vi "LS370Monitor_Standalone.vi"() -> ()   [LabVIEW 2016]
uses:
  Instrument_Setup.vi
  Global/Global Variables/global.vi
  Global/Global Variables/Data_Display_global.vi
panel:
  out "MC Temperature":dbl
  out "Still Temperature":dbl
  out "Sorb Temperature (K)":dbl
  in  "Activate Tsweep":bool
  in  "Rate (K/min)":dbl
  in  "Setpoint - Manual":dbl
  out "Setpoint":dbl
  in  "Disable Heater":bool
  out "Tsweeps Running":bool
  in  "Update Lakeshore":bool
  out "Temperatures":cluster{timestamp[], dbl[]}[](graph)
  in  "Sorb Heater":bool
  in  "Sorb Power (mW)":dbl
  in  "Still Power (mW)":dbl
  in  "Still Heater":bool
  out "Analog Power":cluster{timestamp[], dbl[]}[](graph)
  out "Heater Power":cluster{timestamp[], dbl[]}(graph)
  in  "Stopp":bool
  out "MC Heater Output":dbl
  # "Manuelle Steuerung"
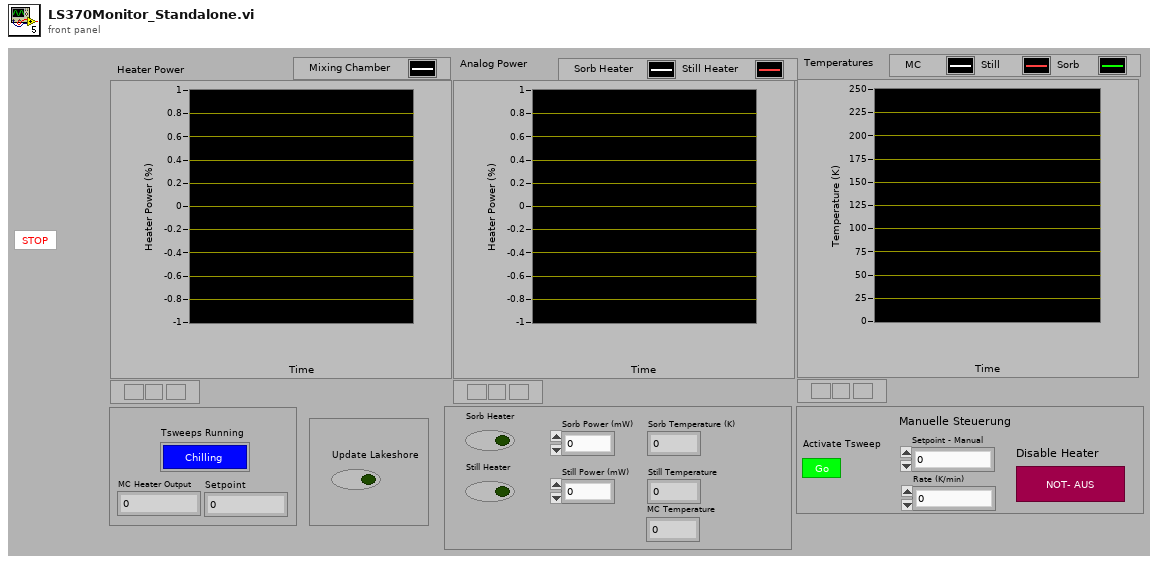
[diagram p1: front panel]
types:
  T1 = cluster{"Control Temperature":dbl[], "Still Temperature":dbl[], "Sorb Temperature":dbl[], "Time":timestamp[], "Analog Out 1 (Sorb)":dbl[], "Analog Out 2 (Still)":dbl[], "MC Heater":dbl[]}
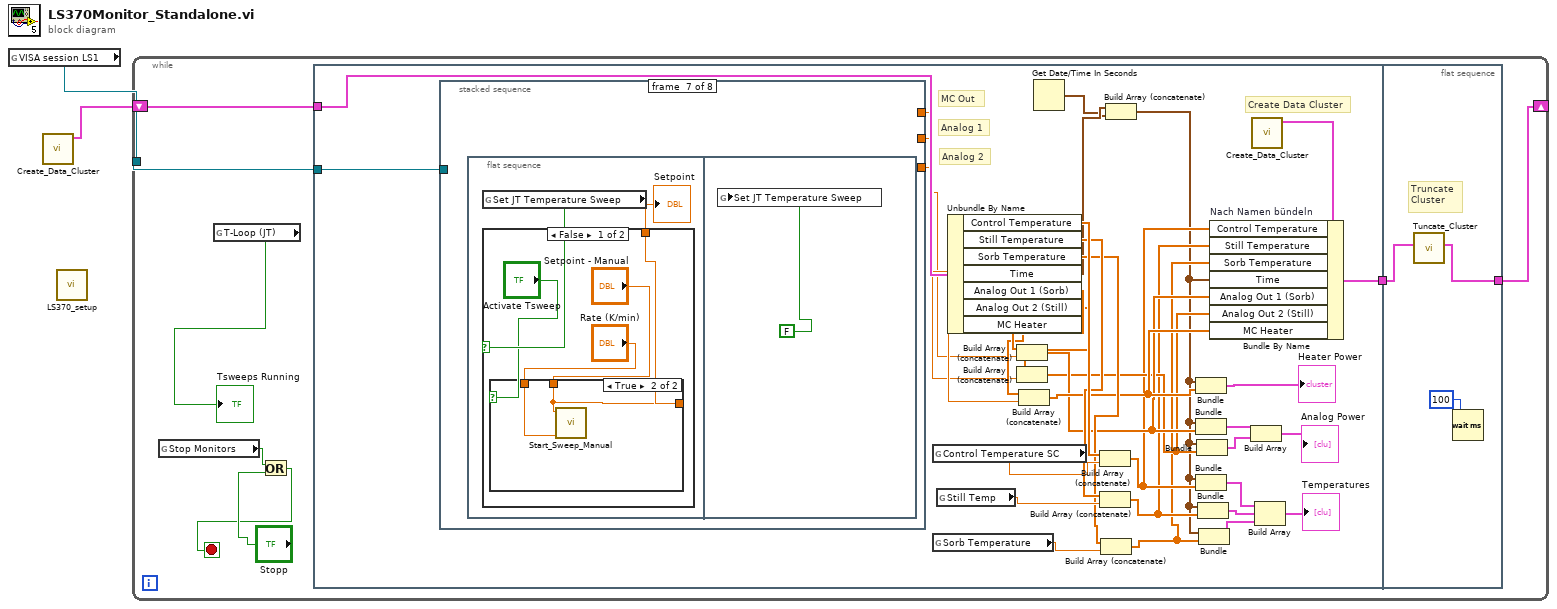
[diagram p0: block diagram]
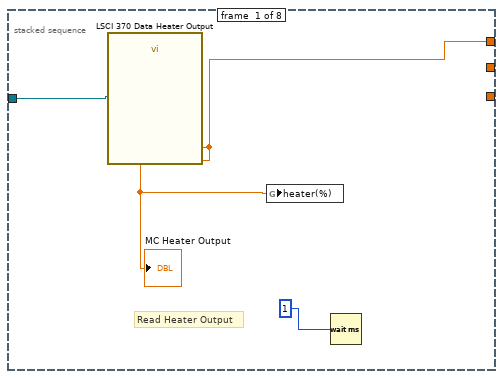
[diagram p2: hidden frame]
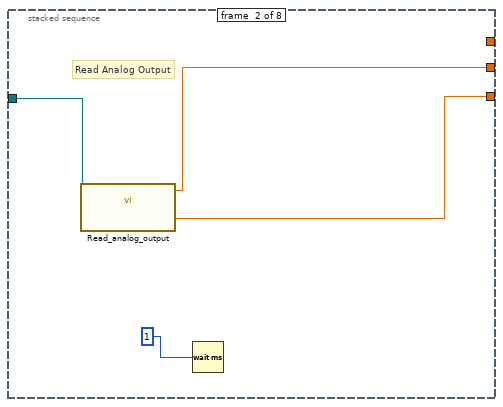
[diagram p3: hidden frame]
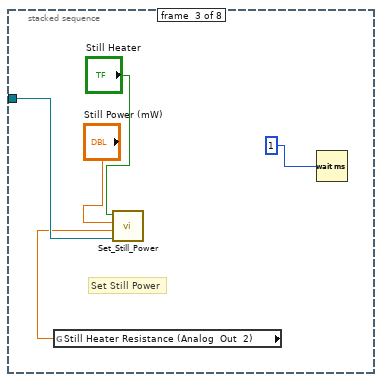
[diagram p4: hidden frame]
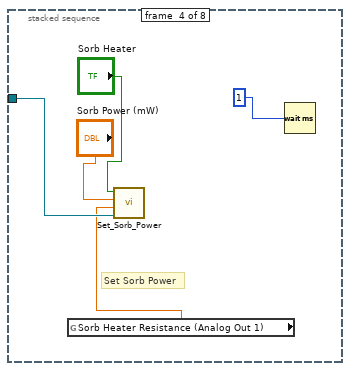
[diagram p5: hidden frame]
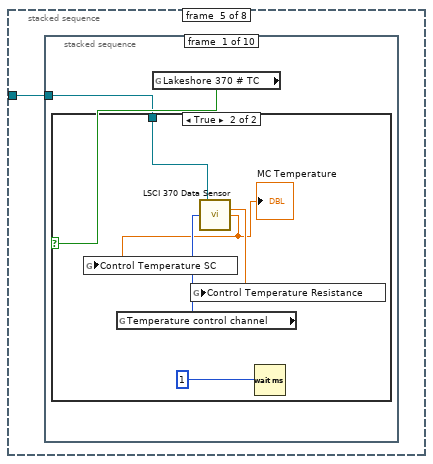
[diagram p6: hidden frame]
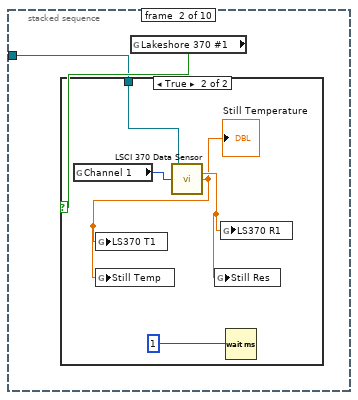
[diagram p8: hidden frame]
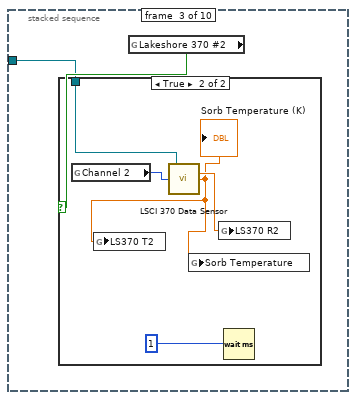
[diagram p10: hidden frame]
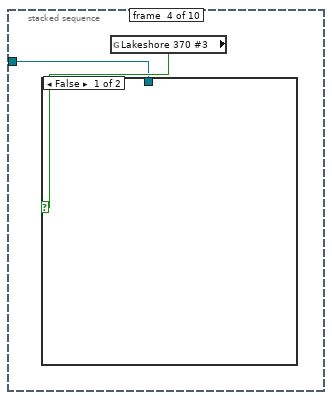
[diagram p12: hidden frame]
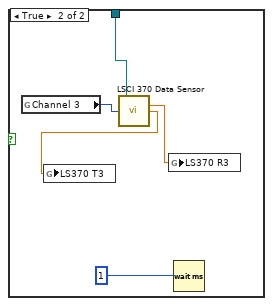
[diagram p13: hidden frame]
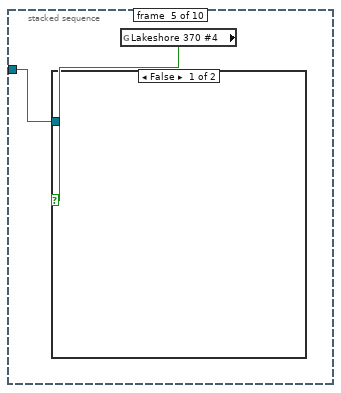
[diagram p14: hidden frame]
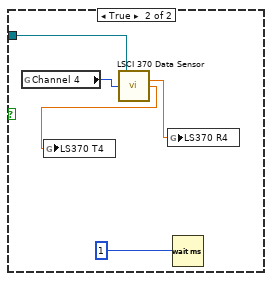
[diagram p15: hidden frame]
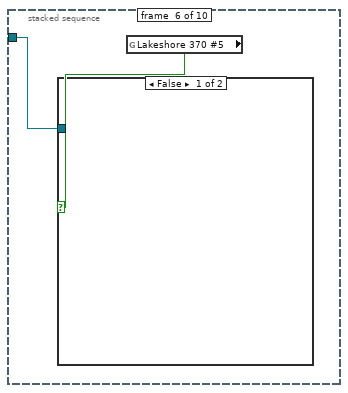
[diagram p16: hidden frame]
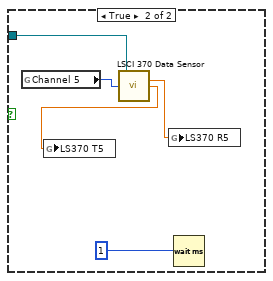
[diagram p17: hidden frame]
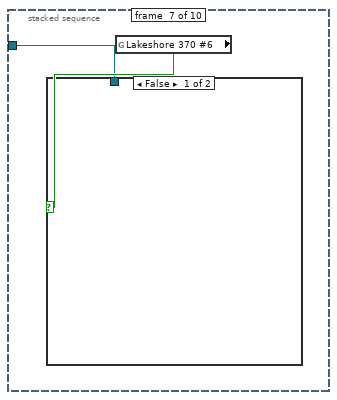
[diagram p18: hidden frame]
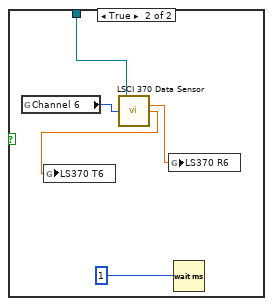
[diagram p19: hidden frame]
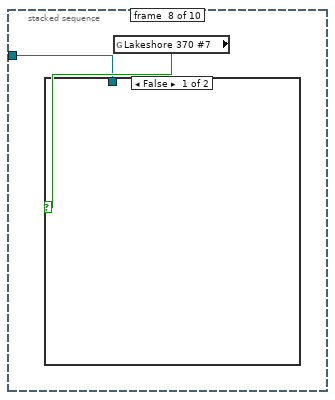
[diagram p20: hidden frame]
diagram:
  n1 = global read "Instrument_Setup.vi" "VISA session LS1"() -> (w2:refnum<visa-resource-name>)
  n2 = call "Create_Data_Cluster.vi"() -> ("Cluster"=w1:T1)  [unwired: 11 in]
  n3 = call "LS370_setup.vi"() -> ()  [unwired: 1 in]
  n4 = while {
    tunnel: w2 -> [w10]
    shift-right: [w6] -> _
    shift-left: w1 -> [w9]
    stop <- w3 stop-if-true
    n5 = global read "Data_Display_global.vi" "Stop Monitors"() -> (w5:bool)
    n6 = global read "global.vi" "T-Loop (JT)"() -> (→"Tsweeps Running":bool)
    n7 = Or(x=w5, y="Stopp") -> (x .or. y?=w3:bool)
    n8 = flat-sequence {
      tunnel: w10 -> [w43]
      tunnel: w9 -> [w40]
      tunnel: [w42] -> w8
      tunnel: [w158] -> w6
      tunnel: w8 -> [w159]
      frame #0 {
        # "Create Data Cluster"
        # "Analog 2"
        # "Analog 1"
        # "MC Out"
        n9 = stacked-sequence {
          tunnel: w43 -> [w46 w50 w53 w58 w61 _ _ _]
          tunnel: [_ w49 _ _ _ _ _ _] -> w25
          tunnel: [_ w48 _ _ _ _ _ _] -> w24
          tunnel: [w45 _ _ _ _ _ _ _] -> w26
          frame #0 {
            # "Read Heater Output"
            n10 = call "LSCI 370 Data Heater Output.vi"("VISA session"=w46) -> ("Heater Output"=w45:dbl)  [unwired: 12 in, 2 out]
            "MC Heater Output" <- w45
            n11 = global write "Data_Display_global.vi" "heater(%)"(w45) -> ()
            n12 = Wait (ms)(milliseconds to wait=1) -> ()  [unwired: 1 out]
          }
          frame #1 {
            # "Read Analog Output"
            n13 = call "Read_analog_output.vi"("VISA session"=w50) -> ("Still Output"=w48:dbl, "Analog Output"=w49:dbl)  [unwired: 9 in]
            n14 = Wait (ms)(milliseconds to wait=1) -> ()  [unwired: 1 out]
          }
          frame #2 {
            # "Set Still Power"
            n15 = global read "Instrument_Setup.vi" "Still Heater Resistance (Analog  Out  2)"() -> (w52:dbl)
            n16 = call "Set_Still_Power.vi"("VISA session"=w53, "Still Heater Resistance (mW)"=w52, "Still Power (mW)"="Still Power (mW)", "Still heater"="Still Heater") -> ()  [unwired: 8 in]
            n17 = Wait (ms)(milliseconds to wait=1) -> ()  [unwired: 1 out]
          }
          frame #3 {
            # "Set Sorb Power"
            n18 = global read "Instrument_Setup.vi" "Sorb Heater Resistance (Analog Out 1)"() -> (w57:dbl)
            n19 = call "Set_Sorb_Power.vi"("VISA session"=w58, "Sorb Heater Resistance (Ohm)"=w57, "Sorb Power (mW)"="Sorb Power (mW)", "Sorb heater"="Sorb Heater") -> ()  [unwired: 8 in]
            n20 = Wait (ms)(milliseconds to wait=1) -> ()  [unwired: 1 out]
          }
          frame #4 {
            n21 = stacked-sequence {
              tunnel: w61 -> [w62 w69 w76 w83 w90 w97 w104 w111 w118 w125]
              frame #0 {
                n22 = global read "Instrument_Setup.vi" "Lakeshore 370 # TC"() -> (w63:bool)
                n23 = case shown="True" w63 {
                  tunnel: w62 -> [_ w65]
                  frame False {
                  }
                  frame True {
                    n24 = global read "Instrument_Setup.vi" "Temperature control channel"() -> (w68:i32)
                    n25 = call "LSCI 370 Data Sensor.vi"("VISA session"=w65, "Channel (1)"=w68) -> ("Resistance Reading"=w66:dbl, "Kelvin Reading"=w64:dbl)  [unwired: 9 in, 3 out]
                    "MC Temperature" <- w64
                    n26 = global write "Data_Display_global.vi" "Control Temperature SC"(w64) -> ()
                    n27 = global write "Data_Display_global.vi" "Control Temperature Resistance"(w66) -> ()
                    n28 = Wait (ms)(milliseconds to wait=1) -> ()  [unwired: 1 out]
                  }
                }
              }
              frame #1 {
                n29 = global read "Instrument_Setup.vi" "Lakeshore 370 #1"() -> (w70:bool)
                n30 = case shown="True" w70 {
                  tunnel: w69 -> [_ w73]
                  frame False {
                  }
                  frame True {
                    n31 = global read "Instrument_Setup.vi" "Channel 1"() -> (w75:i32)
                    n32 = call "LSCI 370 Data Sensor.vi"("VISA session"=w73, "Channel (1)"=w75) -> ("Resistance Reading"=w72:dbl, "Kelvin Reading"=w71:dbl)  [unwired: 9 in, 3 out]
                    "Still Temperature" <- w71
                    n33 = global write "Data_Display_global.vi" "LS370 T1"(w71) -> ()
                    n34 = global write "Data_Display_global.vi" "Still Temp"(w71) -> ()
                    n35 = global write "Data_Display_global.vi" "Still Res"(w72) -> ()
                    n36 = global write "Data_Display_global.vi" "LS370 R1"(w72) -> ()
                    n37 = Wait (ms)(milliseconds to wait=1) -> ()  [unwired: 1 out]
                  }
                }
              }
              frame #2 {
                n38 = global read "Instrument_Setup.vi" "Lakeshore 370 #2"() -> (w77:bool)
                n39 = case shown="True" w77 {
                  tunnel: w76 -> [_ w79]
                  frame False {
                  }
                  frame True {
                    n40 = global read "Instrument_Setup.vi" "Channel 2"() -> (w82:i32)
                    n41 = call "LSCI 370 Data Sensor.vi"("VISA session"=w79, "Channel (1)"=w82) -> ("Resistance Reading"=w80:dbl, "Kelvin Reading"=w78:dbl)  [unwired: 9 in, 3 out]
                    "Sorb Temperature (K)" <- w78
                    n42 = global write "Data_Display_global.vi" "LS370 T2"(w78) -> ()
                    n43 = global write "Data_Display_global.vi" "Sorb Temperature"(w78) -> ()
                    n44 = global write "Data_Display_global.vi" "LS370 R2"(w80) -> ()
                    n45 = Wait (ms)(milliseconds to wait=1) -> ()  [unwired: 1 out]
                  }
                }
              }
              frame #3 {
                n46 = global read "Instrument_Setup.vi" "Lakeshore 370 #3"() -> (w84:bool)
                n47 = case shown="False" w84 {
                  tunnel: w83 -> [_ w85]
                  frame False {
                  }
                  frame True {
                    n48 = global read "Instrument_Setup.vi" "Channel 3"() -> (w89:i32)
                    n49 = call "LSCI 370 Data Sensor.vi"("VISA session"=w85, "Channel (1)"=w89) -> ("Resistance Reading"=w86:dbl, "Kelvin Reading"=w87:dbl)  [unwired: 9 in, 3 out]
                    n50 = global write "Data_Display_global.vi" "LS370 T3"(w87) -> ()
                    n51 = global write "Data_Display_global.vi" "LS370 R3"(w86) -> ()
                    n52 = Wait (ms)(milliseconds to wait=1) -> ()  [unwired: 1 out]
                  }
                }
              }
              frame #4 {
                n53 = global read "Instrument_Setup.vi" "Lakeshore 370 #4"() -> (w91:bool)
                n54 = case shown="False" w91 {
                  tunnel: w90 -> [_ w92]
                  frame False {
                  }
                  frame True {
                    n55 = global read "Instrument_Setup.vi" "Channel 4"() -> (w96:i32)
                    n56 = call "LSCI 370 Data Sensor.vi"("VISA session"=w92, "Channel (1)"=w96) -> ("Resistance Reading"=w93:dbl, "Kelvin Reading"=w94:dbl)  [unwired: 9 in, 3 out]
                    n57 = global write "Data_Display_global.vi" "LS370 T4"(w94) -> ()
                    n58 = global write "Data_Display_global.vi" "LS370 R4"(w93) -> ()
                    n59 = Wait (ms)(milliseconds to wait=1) -> ()  [unwired: 1 out]
                  }
                }
              }
              frame #5 {
                n60 = global read "Instrument_Setup.vi" "Lakeshore 370 #5"() -> (w98:bool)
                n61 = case shown="False" w98 {
                  tunnel: w97 -> [_ w99]
                  frame False {
                  }
                  frame True {
                    n62 = global read "Instrument_Setup.vi" "Channel 5"() -> (w103:i32)
                    n63 = call "LSCI 370 Data Sensor.vi"("VISA session"=w99, "Channel (1)"=w103) -> ("Resistance Reading"=w100:dbl, "Kelvin Reading"=w101:dbl)  [unwired: 9 in, 3 out]
                    n64 = global write "Data_Display_global.vi" "LS370 T5"(w101) -> ()
                    n65 = global write "Data_Display_global.vi" "LS370 R5"(w100) -> ()
                    n66 = Wait (ms)(milliseconds to wait=1) -> ()  [unwired: 1 out]
                  }
                }
              }
              frame #6 {
                n67 = global read "Instrument_Setup.vi" "Lakeshore 370 #6"() -> (w105:bool)
                n68 = case shown="False" w105 {
                  tunnel: w104 -> [_ w106]
                  frame False {
                  }
                  frame True {
                    n69 = global read "Instrument_Setup.vi" "Channel 6"() -> (w110:i32)
                    n70 = call "LSCI 370 Data Sensor.vi"("VISA session"=w106, "Channel (1)"=w110) -> ("Resistance Reading"=w107:dbl, "Kelvin Reading"=w108:dbl)  [unwired: 9 in, 3 out]
                    n71 = global write "Data_Display_global.vi" "LS370 T6"(w108) -> ()
                    n72 = global write "Data_Display_global.vi" "LS370 R6"(w107) -> ()
                    n73 = Wait (ms)(milliseconds to wait=1) -> ()  [unwired: 1 out]
                  }
                }
              }
              frame #7 {
                n74 = global read "Instrument_Setup.vi" "Lakeshore 370 #7"() -> (w112:bool)
                n75 = case shown="False" w112 {
                  tunnel: w111 -> [_ w113]
                  frame False {
                  }
                  frame True {
                    n76 = global read "Instrument_Setup.vi" "Channel 7"() -> (w117:i32)
                    n77 = call "LSCI 370 Data Sensor.vi"("VISA session"=w113, "Channel (1)"=w117) -> ("Resistance Reading"=w114:dbl, "Kelvin Reading"=w115:dbl)  [unwired: 9 in, 3 out]
                    n78 = global write "Data_Display_global.vi" "LS370 T7"(w115) -> ()
                    n79 = global write "Data_Display_global.vi" "LS370 R7"(w114) -> ()
                    n80 = Wait (ms)(milliseconds to wait=1) -> ()  [unwired: 1 out]
                  }
                }
              }
              frame #8 {
                n81 = global read "Instrument_Setup.vi" "Lakeshore 370 #8"() -> (w119:bool)
                n82 = case shown="False" w119 {
                  tunnel: w118 -> [_ w120]
                  frame False {
                  }
                  frame True {
                    n83 = global read "Instrument_Setup.vi" "Channel 8"() -> (w124:i32)
                    n84 = call "LSCI 370 Data Sensor.vi"("VISA session"=w120, "Channel (1)"=w124) -> ("Resistance Reading"=w121:dbl, "Kelvin Reading"=w122:dbl)  [unwired: 9 in, 3 out]
                    n85 = global write "Data_Display_global.vi" "LS370 T8"(w122) -> ()
                    n86 = global write "Data_Display_global.vi" "LS370 R8"(w121) -> ()
                    n87 = Wait (ms)(milliseconds to wait=1) -> ()  [unwired: 1 out]
                  }
                }
              }
              frame #9 {
                n88 = global read "Instrument_Setup.vi" "Lakeshore 370 #9"() -> (w126:bool)
                n89 = case shown="False" w126 {
                  tunnel: w125 -> [_ w127]
                  frame False {
                  }
                  frame True {
                    n90 = global read "Instrument_Setup.vi" "Channel 9"() -> (w131:i32)
                    n91 = call "LSCI 370 Data Sensor.vi"("VISA session"=w127, "Channel (1)"=w131) -> ("Resistance Reading"=w128:dbl, "Kelvin Reading"=w129:dbl)  [unwired: 9 in, 3 out]
                    n92 = global write "Data_Display_global.vi" "LS370 T9"(w129) -> ()
                    n93 = global write "Data_Display_global.vi" "LS370 R9"(w128) -> ()
                    n94 = Wait (ms)(milliseconds to wait=1) -> ()  [unwired: 1 out]
                  }
                }
              }
            }
          }
          frame #5 {
            n95 = case shown="True" "Update Lakeshore" {
              frame False {
              }
              frame True {
                n96 = flat-sequence {
                  frame #0 {
                    n97 = call "LS370_setup.vi"() -> ()  [unwired: 1 in]
                    n98 = Wait (ms)(milliseconds to wait=1) -> ()  [unwired: 1 out]
                  }
                  frame #1 {
                    n99 = local write "Update Lakeshore"(FALSE) -> ()
                  }
                }
              }
            }
          }
          frame #6 {
            n100 = flat-sequence {
              frame #0 {
                n101 = global read "global.vi" "Set JT Temperature Sweep"() -> (w136:bool)
                n102 = case shown="False" w136 {
                  tunnel: [w137 w149] -> w135
                  frame False {
                    n103 = case shown="True" "Activate Tsweep" {
                      tunnel: "Setpoint - Manual" -> [_ w147]
                      tunnel: "Rate (K/min)" -> [_ w148]
                      tunnel: [w141 w147] -> w137
                      frame False {
                        n104 = global read "global.vi" "Cerrent State"() -> (w144:i32)
                        n105 = Equal?(x=1, y=w144) -> (x = y?=w142:bool)
                        n106 = case shown="False" w142 {
                          tunnel: [w145 w146] -> w141
                          frame False {
                            n107 = global read "global.vi" "T final (K)"() -> (w145:dbl)
                          }
                          frame True {
                            n108 = global read "global.vi" "T init. (K)"() -> (w146:dbl)
                          }
                        }
                      }
                      frame True {
                        n109 = call "Start_Sweep_Manual.vi"("Rate"=w148, "Setpoint"=w147) -> ()  [unwired: 10 in]
                      }
                    }
                  }
                  frame True {
                    n110 = call "Start_Ramping.vi"() -> ("Setpoint"=w149:dbl)  [unwired: 11 in]
                    n111 = Wait (ms)(milliseconds to wait=1) -> ()  [unwired: 1 out]
                  }
                }
                "Setpoint" <- w135
              }
              frame #1 {
                n112 = global write "global.vi" "Set JT Temperature Sweep"(FALSE) -> ()
              }
            }
          }
          frame #7 {
            n113 = flat-sequence {
              frame #0 {
                n114 = Or(x=FALSE, y="Disable Heater") -> (x .or. y?=w154:bool)
                n115 = case shown="True" w154 {
                  frame False {
                  }
                  frame True {
                    n116 = call "Disable_Zone_Tuning.vi"() -> ()  [unwired: 1 in]
                    n117 = Wait (ms)(milliseconds to wait=1) -> ()  [unwired: 1 out]
                  }
                }
              }
              frame #1 {
                n118 = global write "global.vi" "Disable Zone Tuning"(FALSE) -> ()
              }
            }
          }
        }
        n119 = global read "Data_Display_global.vi" "Control Temperature SC"() -> (w37:dbl)
        n120 = global read "Data_Display_global.vi" "Sorb Temperature"() -> (w34:dbl)
        n121 = global read "Data_Display_global.vi" "Still Temp"() -> (w36:dbl)
        n122 = Unbundle By Name(w40) -> ("Control Temperature"=w39:dbl[], "Still Temperature"=w38:dbl[], "Sorb Temperature"=w35:dbl[], "Time"=w12:timestamp[], "Analog Out 1 (Sorb)"=w29:dbl[], "Analog Out 2 (Still)"=w28:dbl[], "MC Heater"=w27:dbl[])
        n123 = Build Array (concatenate)(w29, w25) -> (w19:dbl[])
        n124 = Build Array (concatenate)(w28, w24) -> (w18:dbl[])
        n125 = Build Array (concatenate)(w27, w26) -> (w20:dbl[])
        n126 = Get Date/Time In Seconds() -> (seconds since 1Jan1904=w11:timestamp)
        n127 = Build Array (concatenate)(w39, w37) -> (w17:dbl[])
        n128 = Build Array (concatenate)(w38, w36) -> (w16:dbl[])
        n129 = Build Array (concatenate)(w35, w34) -> (w15:dbl[])
        n130 = Build Array (concatenate)(w12, w11) -> (w14:timestamp[])
        n131 = Bundle(w14, w20) -> (→"Heater Power":cluster{timestamp[], dbl[]})  [unwired: 1 in]
        n132 = Bundle(w14, w19) -> (w23:cluster{timestamp[], dbl[]})  [unwired: 1 in]
        n133 = Bundle(w14, w17) -> (w33:cluster{timestamp[], dbl[]})  [unwired: 1 in]
        n134 = Bundle(w14, w18) -> (w22:cluster{timestamp[], dbl[]})  [unwired: 1 in]
        n135 = Bundle(w14, w16) -> (w32:cluster{timestamp[], dbl[]})  [unwired: 1 in]
        n136 = Bundle(w14, w15) -> (w31:cluster{timestamp[], dbl[]})  [unwired: 1 in]
        n137 = Build Array(w23, w22) -> (→"Analog Power":cluster{timestamp[], dbl[]}[])
        n138 = call "Create_Data_Cluster.vi"() -> ("Cluster"=w13:T1)  [unwired: 11 in]
        n139 = Bundle By Name "Nach Namen bündeln"(cluster=w13, "Control Temperature"=w17, "Still Temperature"=w16, "Sorb Temperature"=w15, "Time"=w14, "Analog Out 1 (Sorb)"=w19, "Analog Out 2 (Still)"=w18, "MC Heater"=w20) -> (w42:T1)
        n140 = Build Array(w33, w32, w31) -> (→"Temperatures":cluster{timestamp[], dbl[]}[])
      }
      frame #1 {
        # "Truncate \nCluster"
        n141 = call "Tuncate_Cluster.vi"("Eingangscluster"=w159) -> ("Cluster"=w158:T1)  [unwired: 10 in]
        n142 = Wait (ms)(milliseconds to wait=100) -> ()  [unwired: 1 out]
      }
    }
  }
